vi "Enable RT.vi"(8 "error in":errorcluster, 10 "terminal address":u8=1, 11 "module handle":u32) -> (0 "error out":errorcluster, 3 "module handle out":u32)   [LabVIEW 2020, in "AIM MIL-STD-1553 Hardware API.lvlib"]
uses:
  AIM MIL-STD-1553 Hardware API.lvlib
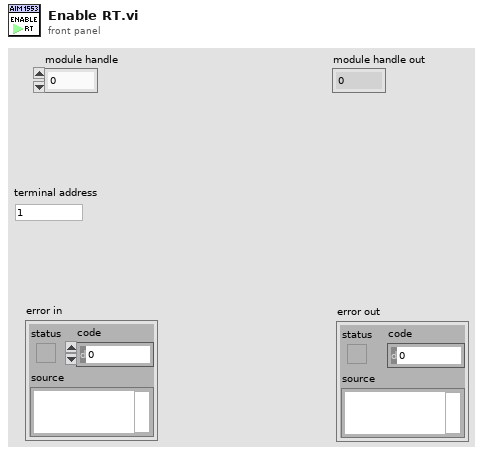
[diagram p1: front panel]
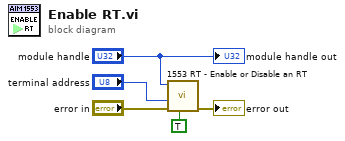
[diagram p0: block diagram]
diagram:
  n1 = call <instrlib>:"1553 RT - Enable or Disable an RT.vi"("Enabled (false)"=TRUE, "Error In (none)"="error in", "RT Address (1)"="terminal address", "Module Handle"="module handle") -> ("Error Out"=→"error out":errorcluster)  [unwired: 7 in]
  "module handle out" <- "module handle"
